vi "SessionManager.vi"() -> ()   [LabVIEW 2010]
uses:
  TimeStamper/TimeStamper.lvclass
  <vilib>/Utility/config.llb/Read Key (I32).vi
  <vilib>/Utility/config.llb/Read Key (Path).vi
  <vilib>/Utility/config.llb/NI_LVConfig.lvlib
panel:
  out "Messages":T1(array[cluster])
  out "Timestamps":T2(array[cluster])
  out "error out":errorcluster
  in  "Experimenter":string(combo)="Unselected"
  out "Session Path":path
  in  "stop":bool
  in  "Subject":string(combo)="Testing"
  in  "Root Path":path=path "M:/"
  in  "Counter Card":tag="Dev1"
  in  "Sample Lines":tag[](array[tag])=["/Dev3/ai/StartTrigger", "/4498_1/ai/StartTrigger"]
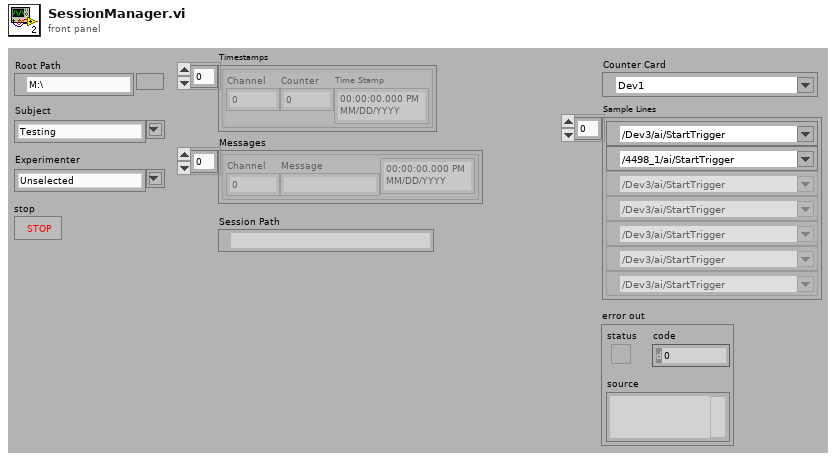
[diagram p1: front panel]
types:
  T1 = cluster{"Channel":dbl, "Message":string, timestamp}[]
  T2 = cluster{"Channel":i32, "Counter":u32, "Time Stamp":timestamp}[]
  T3 = typedef "NI_LVConfig.lvlib/Config Data RefNum.ctl" = refnum<k1>
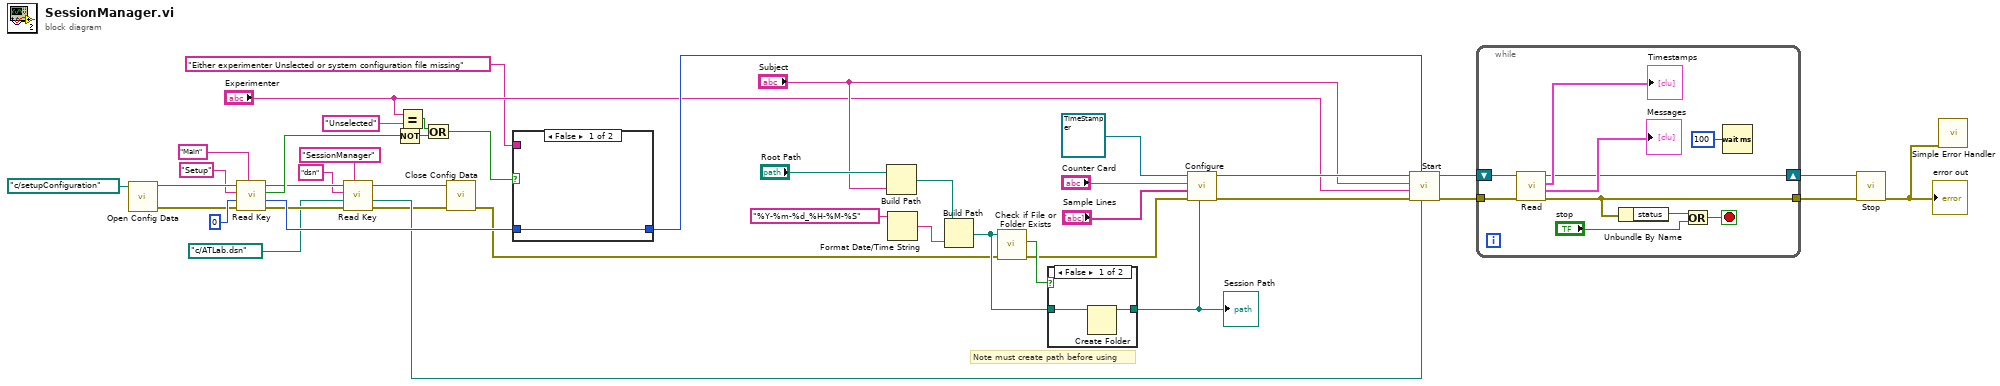
[diagram p0: block diagram]
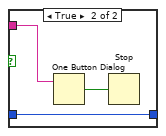
[diagram p2: hidden frame]
diagram:
  # "Note must create path before using"
  n1 = call <vilib>:"Open Config Data.vi"("configuration file path"=path "c:/setupConfiguration") -> ("error out"=w20:errorcluster, "refnum"=w24:T3)  [unwired: 8 in, 1 out]
  n2 = call-poly <vilib>:"Read Key.vi"("section"="Main", "error in (no error)"=w20, "default value"=0, "key"="Setup", "refnum"=w24) -> ("error out"=w7:errorcluster, "value"=w19:i32, "found?"=w14:bool, "refnum out"=w8:T3)  [unwired: 3 in]
  n3 = call-poly <vilib>:"Read Key.vi"("section"="SessionManager", "error in (no error)"=w7, "default value"=path "c:/ATLab.dsn", "key"="dsn", "refnum"=w8) -> ("error out"=w3:errorcluster, "value"=w4:path, "refnum out"=w2:T3)  [unwired: 3 in, 1 out]
  n4 = Not(x=w14) -> (.not. x?=w13:bool)
  n5 = Equal?(x="Experimenter", y="Unselected") -> (x = y?=w12:bool)
  n6 = Or(x=w12, y=w13) -> (x .or. y?=w11:bool)
  n7 = call <vilib>:"Close Config Data.vi"("error in (no error)"=w3, "refnum"=w2) -> ("error out"=w17:errorcluster)  [unwired: 8 in, 1 out]
  n8 = case shown="False" w11 {
    tunnel: w19 -> [w44 w47]
    tunnel: [w44 w47] -> w18
    tunnel: "Either experimenter Unslected or system configuration file missing" -> [_ w46]
    frame False {
    }
    frame True {
      n9 = One Button Dialog(message=w46) -> (true=w45:bool)  [unwired: 1 in]
      n10 = Stop(stop? (T)=w45) -> ()
    }
  }
  n11 = Build Path(base path="Root Path", name or relative path="Subject") -> (appended path=w38:path)
  n12 = Format Date/Time String(time format string (%c)="%Y-%m-%d_%H-%M-%S") -> (date/time string=w34:string)  [unwired: 2 out]
  n13 = Build Path(base path=w38, name or relative path=w34) -> (appended path=w33:path)
  n14 = call <vilib>:"Check if File or Folder Exists.vi"("error in (no error)"=w17, "path"=w33) -> ("error out"=w27:errorcluster, "file or folder exists?"=w37:bool)  [unwired: 8 out]
  n15 = case shown="False" w37 {
    tunnel: w33 -> [w49 w50]
    tunnel: [w48 w50] -> w32
    frame False {
      n16 = Create Folder(path (use dialog)=w49) -> (created path=w48:path)  [unwired: 2 in, 2 out]
    }
    frame True {
    }
  }
  "Session Path" <- w32
  n17 = call-dynamic "Configure.vi"("Session Path"=w32, "error in (no error)"=w27, "Sample Lines"="Sample Lines", "DAQmx Device Name"="Counter Card", "TimeStamper in"=refnum<class "TimeStamper.lvclass"> refnum ("TimeStamper.lvclass")) -> ("error out"=w41:errorcluster, "TimeStamper out"=w42:refnum<class "TimeStamper.lvclass">)  [unwired: 5 in]
  n18 = call-dynamic "Start.vi"("connection dsn"=w4, "setup"=w18, "error in (no error)"=w41, "experimenter"="Experimenter", "subject"="Subject", "TimeStamper in"=w42) -> ("error out"=w31:errorcluster, "TimeStamper out"=w30:refnum<class "TimeStamper.lvclass">)  [unwired: 4 in]
  n19 = while {
    tunnel: w31 -> [w58]
    shift-right: [w56] -> w29
    shift-left: w30 -> [w57]
    tunnel: [w54] -> w28
    stop <- w51 stop-if-true
    n20 = call-dynamic "Read.vi"("error in (no error)"=w58, "TimeStamper in"=w57) -> ("error out"=w54:errorcluster, "Messages"=→"Messages":T1, "Timestamps"=→"Timestamps":T2, "TimeStamper out"=w56:refnum<class "TimeStamper.lvclass">)  [unwired: 6 in]
    n21 = Unbundle By Name(w54) -> ("status"=w53:bool)
    n22 = Or(x=w53, y="stop") -> (x .or. y?=w51:bool)
    n23 = Wait (ms)(milliseconds to wait=u32 100) -> ()  [unwired: 1 out]
  }
  n24 = call-dynamic "Stop.vi"("error in (no error)"=w28, "TimeStamper in"=w29) -> ("error out"=w9:errorcluster)  [unwired: 8 in, 1 out]
  "error out" <- w9
  n25 = call <vilib>:"Simple Error Handler.vi"("error in (no error)"=w9) -> ()  [unwired: 4 in, 5 out]
